vi "findAndTargetNeurons.vi"() -> ()   [LabVIEW 2017]
uses:
  globalUtilities.vi
  globalDevices.vi
  <userlib>/Hamamatsu Video Capture/tm_getframe16_40.vi
panel:
  out "projected volume":u64[][](graph)
  in  "index (vol)":i32
  in  "targetNeuron":i32[](array[numeric])=[24, 23, 15]
  in  "stop":bool
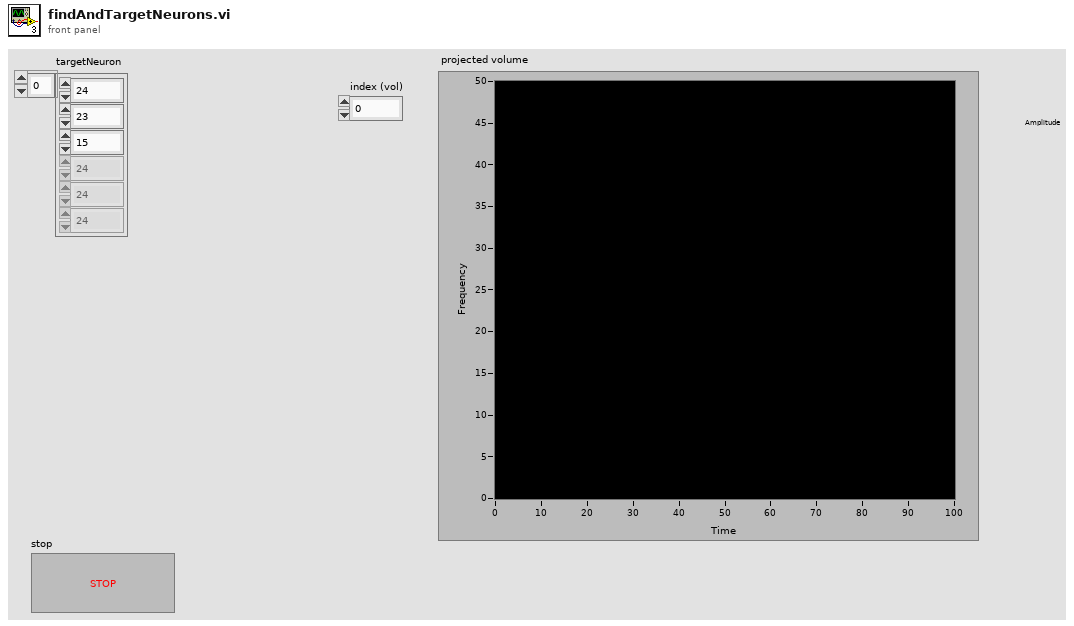
[diagram p1: front panel]
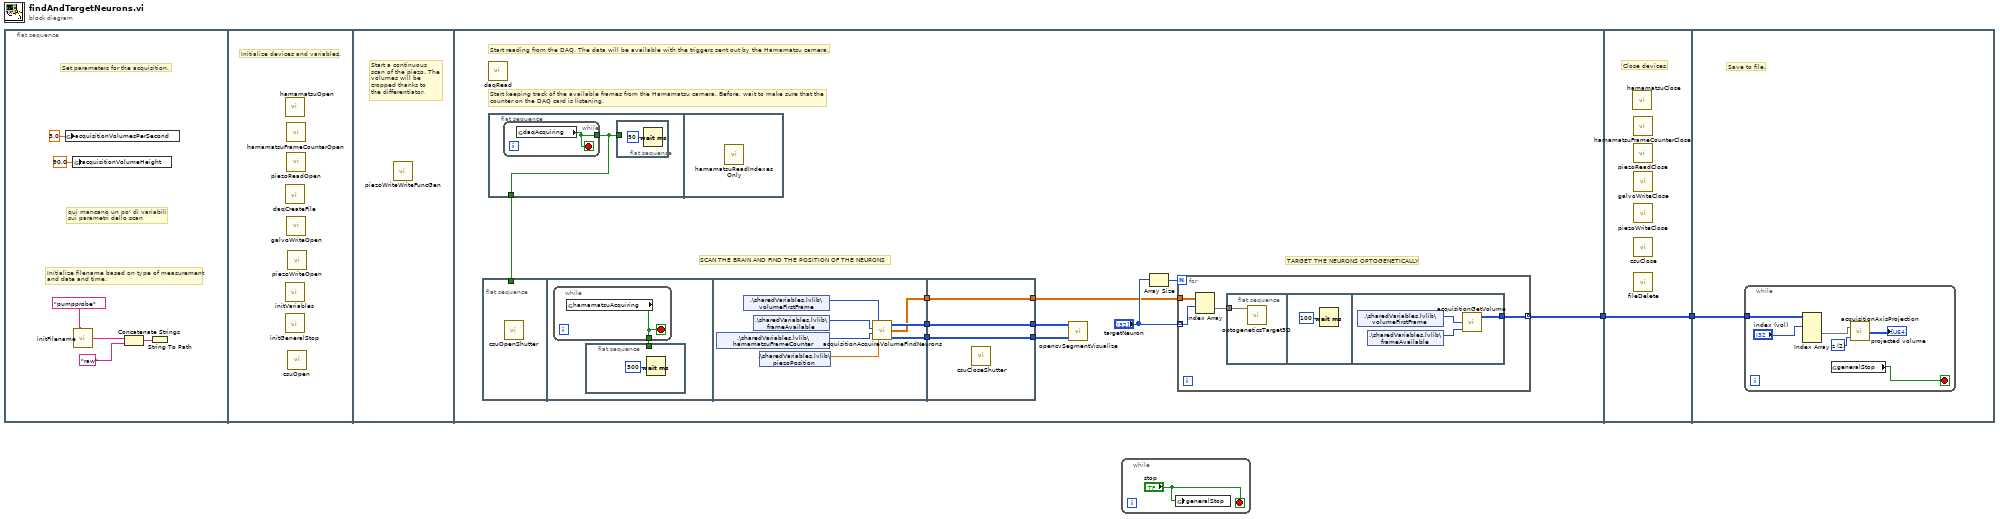
[diagram p0: block diagram]
diagram:
  n1 = flat-sequence {
    tunnel: [w13] -> w1
    tunnel: [w44] -> w2
    tunnel: w1 -> [w44]
    tunnel: w2 -> [w45]
    frame #0 {
      # "Initialize filename based on type of measurement\nand date and time."
      # "qui mancano un po' di variabili\nsui parametri dello scan"
      # "Set parameters for the acquisition."
      n2 = global write "globalUtilities.vi" "acquisitionVolumesPerSecond"(3.0 ("acquisitionVolumesPerSecond")) -> ()
      n3 = global write "globalUtilities.vi" "acquisitionVolumeHeight"(90.0 ("acquisitionVolumeHeight")) -> ()
      n4 = call "initFilename.vi"("Experiment type"="pumpprobe") -> ("folder name"=w3:string)  [unwired: 1 in]
      n5 = Concatenate Strings(w3, "raw") -> (w4:string)
      n6 = String To Path(string=w4) -> ()  [unwired: 1 out]
    }
    frame #1 {
      # "Initialize devices and variables."
      n7 = call "initVariables.vi"() -> ()  [unwired: 12 in]
      n8 = call "hamamatsuOpen.vi"() -> ()  [unwired: 4 out]
      n9 = call "daqCreateFile.vi"() -> ()  [unwired: 12 in]
      n10 = call "initGeneralStop.vi"() -> ()  [unwired: 1 in]
      n11 = call "hamamatsuFrameCounterOpen.vi"() -> ()  [unwired: 12 in]
      n12 = call "piezoReadOpen.vi"() -> ()  [unwired: 6 in]
      n13 = call "galvoWriteOpen.vi"() -> ()  [unwired: 12 in]
      n14 = call "piezoWriteOpen.vi"() -> ()  [unwired: 2 in]
      n15 = call "csuOpen.vi"() -> ()  [unwired: 14 in, 2 out]
    }
    frame #2 {
      # "Start a continuous\nscan of the piezo. The \nvolumes will be\ncropped thanks to\nthe differentiator."
      n16 = call "piezoWriteWriteFuncGen.vi"() -> ()  [unwired: 12 in]
    }
    frame #3 {
      # "TARGET THE NEURONS OPTOGENETICALLY"
      # "SCAN THE BRAIN AND FIND THE POSITION OF THE NEURONS"
      # "Start keeping track of the available frames from the Hamamatsu camera. Before, wait to make sure that the\ncounter on the DAQ card is listening."
      # "Start reading from the DAQ. The data will be available with the triggers sent out by the Hamamatsu camera."
      n17 = flat-sequence {
        tunnel: w9 -> [_]
        tunnel: [w33] -> w12
        tunnel: [w32] -> w11
        tunnel: [w31] -> w10
        tunnel: [w38] -> w14
        tunnel: [w39] -> w17
        tunnel: [w40] -> w18
        tunnel: w12 -> [w40]
        tunnel: w11 -> [w39]
        tunnel: w10 -> [w38]
        frame #0 {
          n18 = call "csuOpenShutter.vi"() -> ()  [unwired: 16 in]
        }
        frame #1 {
          n19 = while {
            tunnel: [w30] -> w28
            stop <- w30 stop-if-true
            n20 = global read "globalUtilities.vi" "hamamatsuAcquiring"() -> (w30:bool)
          }
          n21 = flat-sequence {
            tunnel: w28 -> [_]
            frame #0 {
              n22 = Wait (ms)(milliseconds to wait=u32 500) -> ()  [unwired: 1 out]
            }
          }
        }
        frame #2 {
          n23 = shared-variable ".\\sharedVariables.lvlib\\hamamatsuFrameCounter"() -> (w35:u32[])  [unwired: 1 in, 1 out]
          n24 = shared-variable ".\\sharedVariables.lvlib\\volumeFirstFrame"() -> (w37:u32[])  [unwired: 1 in, 1 out]
          n25 = shared-variable ".\\sharedVariables.lvlib\\frameAvailable"() -> (w36:i32[])  [unwired: 1 in, 1 out]
          n26 = shared-variable ".\\sharedVariables.lvlib\\piezoPosition"() -> (w34:dbl[])  [unwired: 1 in, 1 out]
          n27 = call "acquisitionAcquireVolumeFindNeurons.vi"("piezoPosition"=w34, "hamamatsuFrameCounter"=w35, "frameAvailable"=w36, "volumeFirstFrame"=w37) -> ("XY"=w32:u16[][][], "XYZ"=w31:dbl[][], "volume out"=w33:u16[][][])
        }
        frame #3 {
          n28 = call "csuCloseShutter.vi"() -> ()  [unwired: 16 in]
        }
      }
      n29 = call "daqRead.vi"() -> ()  [unwired: 3 in]
      n30 = flat-sequence {
        tunnel: [w41] -> w9
        frame #0 {
          n31 = while {
            tunnel: [w43] -> w41
            stop <- w43 stop-if-true
            n32 = global read "globalUtilities.vi" "daqAcquiring"() -> (w43:bool)
          }
          n33 = flat-sequence {
            tunnel: w41 -> [_]
            frame #0 {
              n34 = Wait (ms)(milliseconds to wait=u32 50) -> ()  [unwired: 1 out]
            }
          }
        }
        frame #1 {
          n35 = call "hamamatsuReadIndexesOnly.vi"() -> ()  [unwired: 12 in]
        }
      }
      n36 = call "opencvSegmentVisualize.vi"("XY"=w17, "ImgIn"=w18) -> ()  [unwired: 1 in]
      n37 = Array Size(array="targetNeuron") -> (size(s)=w16:i32)
      n38 = for {
        N: w16 -> [_]
        tunnel: w14 -> [w22]
        tunnel: "targetNeuron" -> [w21] mode=indexing
        tunnel: [w19] -> w13 mode=indexing
        n39 = Index Array(array=w22, index (row)=w21) -> (element=w20:dbl[])  [unwired: 1 in]
        n40 = flat-sequence {
          tunnel: w20 -> [w23]
          tunnel: [w25] -> w19
          frame #0 {
            n41 = call "optogeneticsTarget3D.vi"("xyz"=w23) -> ()  [unwired: 4 in]
          }
          frame #1 {
            n42 = Wait (ms)(milliseconds to wait=u32 100) -> ()  [unwired: 1 out]
          }
          frame #2 {
            n43 = shared-variable ".\\sharedVariables.lvlib\\volumeFirstFrame"() -> (w27:u32[])  [unwired: 1 in, 1 out]
            n44 = shared-variable ".\\sharedVariables.lvlib\\frameAvailable"() -> (w26:i32[])  [unwired: 1 in, 1 out]
            n45 = call "acquisitionGetVolume.vi"("frameAvailable"=w26, "volumeFirstFrame"=w27) -> ("volume out"=w25:u16[][][])  [unwired: 1 in, 2 out]
          }
        }
      }
    }
    frame #4 {
      # "Close devices."
      n46 = call "hamamatsuClose.vi"() -> ()  [unwired: 1 out]
      n47 = call "hamamatsuFrameCounterClose.vi"() -> ()  [unwired: 12 in]
      n48 = call "piezoReadClose.vi"() -> ()  [unwired: 1 in]
      n49 = call "galvoWriteClose.vi"() -> ()  [unwired: 12 in]
      n50 = call "piezoWriteClose.vi"() -> ()  [unwired: 1 in]
      n51 = call "csuClose.vi"() -> ()  [unwired: 12 in]
      n52 = call "fileDelete.vi"() -> ()  [unwired: 12 in]
    }
    frame #5 {
      # "Save to file."
      n53 = while {
        tunnel: w45 -> [w51]
        stop <- w48 stop-if-true
        w46 = u16 2 items=["x", "y", "z"] ("axis (z)")
        n54 = Index Array(array=w51, index (dim 0)="index (vol)") -> (element=w47:u16[][][])  [unwired: 3 in]
        n55 = global read "globalUtilities.vi" "generalStop"() -> (w48:bool)
        n56 = call "acquisitionAxisProjection.vi"("axis (z)"=w46, "z stack"=w47) -> ("projected img"=→"projected volume":u64[][])
      }
    }
  }
  n57 = while {
    stop <- "stop" stop-if-true
    n58 = global write "globalUtilities.vi" "generalStop"("stop") -> ()
  }
